vi "Rudder.vi"() -> ()   [LabVIEW 2011]
panel:
  in  "Rudder":dbl
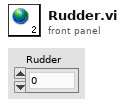
[diagram p1: front panel]
diagram:
